vi "4_3.vi"() -> ()   [LabVIEW 2017]
panel:
  out "Data 3":i32
  out "Data 4":i32
  out "Data 2":i32
  out "Data 1":i32
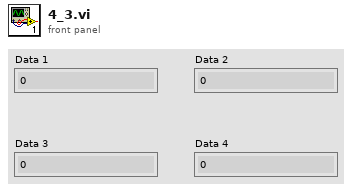
[diagram p1: front panel]
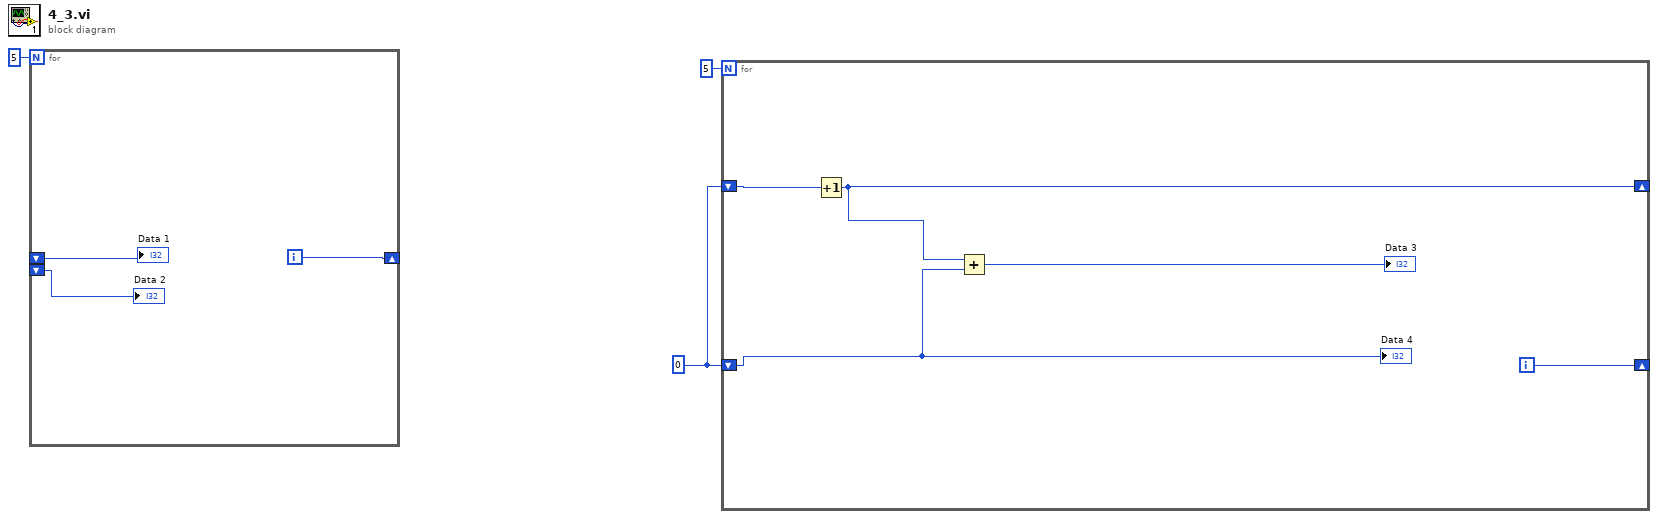
[diagram p0: block diagram]
diagram:
  w2 = 0
  n1 = for {
    N: 5 -> [_]
    shift-right: [w6] -> _
    shift-left: _ -> [w5]
    shift-left: _ -> [w4]
    i -> [w6]
    "Data 1" <- w5
    "Data 2" <- w4
  }
  n2 = for {
    N: 5 -> [_]
    shift-right: [w8] -> _
    shift-left: w2 -> [w10]
    shift-right: [w11] -> _
    shift-left: w2 -> [w7]
    i -> [w11]
    n3 = Increment(x=w10) -> (x+1=w8:i32)
    n4 = Add(x=w8, y=w7) -> (x+y=→"Data 3":i32)
    "Data 4" <- w7
  }
